vi "Associate Instruments to Paths.vi"(0 "Path Groups in":refnum<class "Path Group.lvclass">[](array[class]), 5 "TSM Context":T1, 11 "error in (no error)":errorcluster) -> (4 "Path Groups out":refnum<class "Path Group.lvclass">[](array[class]), 15 "error out":errorcluster)   [LabVIEW 2023, in "RFCalAndFixtureCharact.Common.lvlib"]
uses:
  RFCalAndFixtureCharact.Common.lvlib
  <vilib>/NI_TestStand_SemiconductorModule/NI_TestStand_Semiconductor_Module.lvlibp/PinMap/General/SemiconductorModuleContext.ctl
  Base Classes/Path Group/Path Group.lvclass
  <vilib>/NI_TestStand_SemiconductorModule/NI_TestStand_Semiconductor_Module.lvlibp
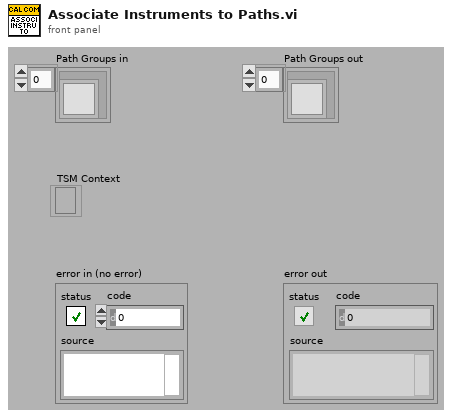
[diagram p1: front panel]
types:
  T1 = typedef "NI_TestStand_Semiconductor_Module.lvlibp/SemiconductorModuleContext.ctl" = refnum<k7>
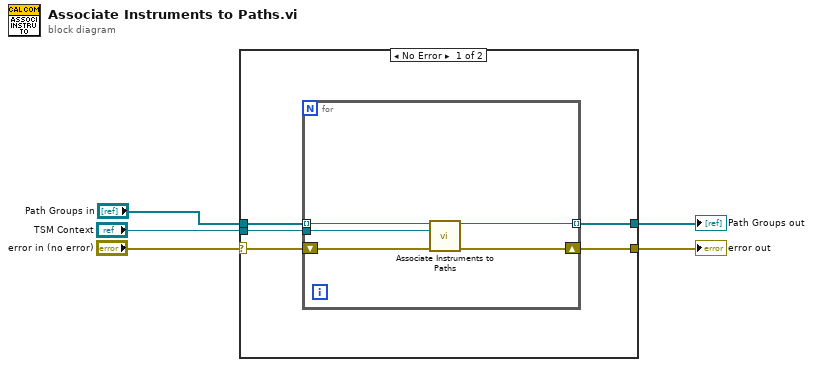
[diagram p0: block diagram]
diagram:
  n1 = case shown="No Error" "error in (no error)" {
    selector: "error in (no error)" -> [w10 w17]
    tunnel: "TSM Context" -> [w9 _]
    tunnel: [w8 w17] -> w3
    tunnel: [w7 w16] -> w2
    tunnel: "Path Groups in" -> [w6 w16]
    frame No Error {
      n2 = for {
        tunnel: w9 -> [w13]
        tunnel: [w12] -> w7 mode=indexing
        shift-right: [w14] -> w8
        shift-left: w10 -> [w15]
        tunnel: w6 -> [w11] mode=indexing
        n3 = call-dynamic "Associate Instruments to Paths.vi"("Path Group in"=w11, "TSM Context"=w13, "error in (no error)"=w15) -> ("Path Group out"=w12:refnum<class "Path Group.lvclass">, "error out"=w14:errorcluster)  [unwired: 11 in]
      }
    }
    frame Error {
    }
  }
  "error out" <- w3
  "Path Groups out" <- w2
